vi "Process.vi"(8 "error in":errorcluster, 11 "DisplayWaveforms":refnum<class "DisplayWaveforms.lvclass">) -> (0 "error out":errorcluster, 3 "DisplayWaveforms out":refnum<class "DisplayWaveforms.lvclass">)   [LabVIEW 2020, in "DisplayWaveform.lvlib" / "DisplayWaveforms.lvclass"]
doc: "Displays all the waveforms using charts."
uses:
  DisplayWaveforms.lvclass
  C:/Program Files (x86)/National Instruments/LabVIEW 2020/vi.lib/JKI/JKI SMO/SMO/SMO.lvclass
  C:/Program Files (x86)/National Instruments/LabVIEW 2020/vi.lib/JKI/JKI SMO/SMO.UI/SMO.UI.lvclass
  <vilib>/JKI/JKI SMO/SMO/Typedefs/Parent Call--Enum.ctl
  Controller/TypeDefs/ChartParamsCluster.ctl
  DisplayWaveforms.lvclass/DisplayWaveforms.ctl
  <vilib>/JKI/JKI SMO/SMO.UI/SMO.UI.lvclass
  <vilib>/JKI/JKI SMO/SMO/SMO.lvclass
panel:
  out "Curr. Sense":dbl[][](graph)
  out "Amp. Volt.":dbl[][](graph)
  out "Ctrl. Eff":dbl[][](graph)
  out "Pos.":dbl[][](graph)
  out "Eddy Volt":dbl[][](graph)
  in  "------------- Registered Events -------------":bool
  in  "------------- Public API -------------":bool
  # "For instructions on how to use the JKI State Machine Objects, examples and video tutorials, visit:\nhttp://jki.net/state-machine-objects/\n\nJKI State Machine Objects™\nhttp://jki.net/state-machine-objects/\nCopyright (C) 2005-2015, JKI <info@jki.net>\nALL RIGHTS RESERVED"
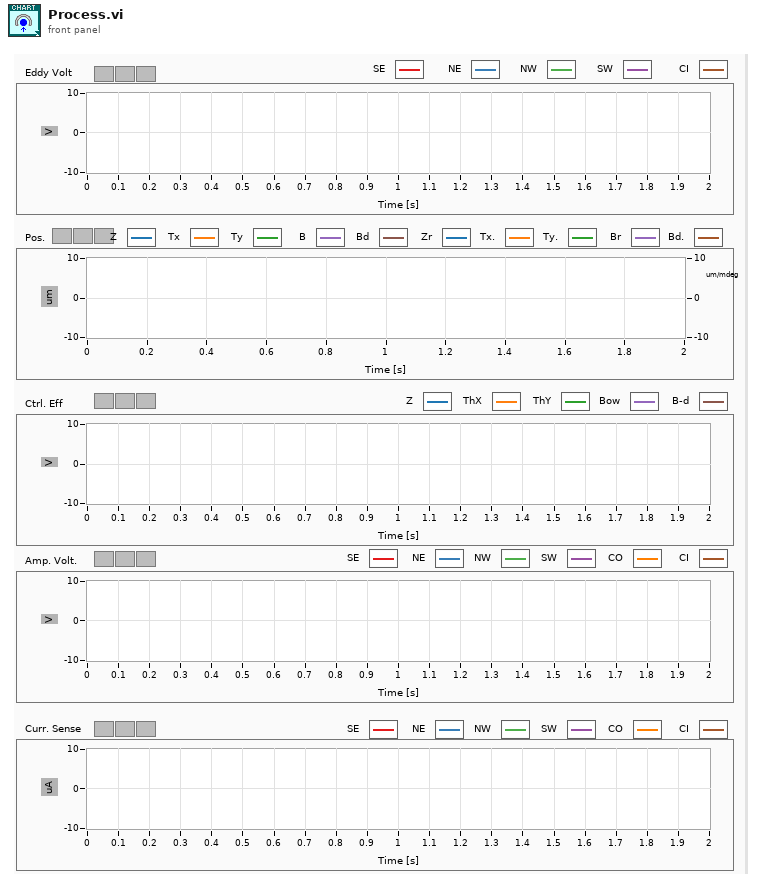
[diagram p1: front panel]
types:
  T1 = typedef "SMO.lvclass/Parent Call--Enum.ctl" = enum16{"Allows parent to run", "Does not request parent to run"}
  T2 = enum32{"invalid app kind", "Development System", "Run Time System", "Student Edition", "Embedded LabVIEW", "Evaluation", "Custom"}
  T3 = enum32{"Invalid", "Standard", "Closed", "Hidden", "Minimized", "Maximized"}
  T4 = typedef "ChartParamsCluster.ctl" = cluster{"Chart ScaleMultipliers":cluster{"WF Xscale Multiplier":dbl, "WF Yscale Multiplier":dbl[]}, "Coord Transform Multipliers":cluster{"Z-Multiplier":dbl, "Th-Multiplier":dbl}}
  T5 = cluster{"Core":cluster{"Current VI Reference":refnum<vi>, "Close Panel on Exit?":bool, "error":errorcluster}, "Self Reference":refnum<class "DisplayWaveforms.lvclass">, "bool":bool, "update chart?":bool, "ChartParams":T4, "Export Folder Path":path}
  T6 = cluster{"Current VI Reference":refnum<vi>, "Close Panel on Exit?":bool, "error":errorcluster}
  T7 = typedef "SMO.lvclass/Protected Events.ctl" = cluster{"StopProcesses":refnum<user-event>, "AbortProcesses":refnum<user-event>, "Config Changed":refnum<user-event>, "Dependency":refnum<user-event>}
  T8 = typedef "DisplayWaveform.lvlib/DisplayWaveforms.lvclass/ProtectedEvents--Cluster.ctl" = cluster{"Clear Chart":refnum<user-event>, "Pause Chart":refnum<user-event>, "Update Chart":refnum<user-event>, "Export Chart":refnum<user-event>, "Set ChartParams":refnum<user-event>}
  T9 = typedef "DisplayWaveform.lvlib/DisplayWaveforms.lvclass/Dependencies--Cluster.ctl" = cluster{"New Value":refnum<user-event>}
  T10 = typedef "imagedata.ctl" = cluster{"image type":i32, "image depth":i32, "image":u8[], "mask":u8[], "colors":u32[], "Rectangle":cluster{"left":i16, "top":i16, "right":i16, "bottom":i16}}
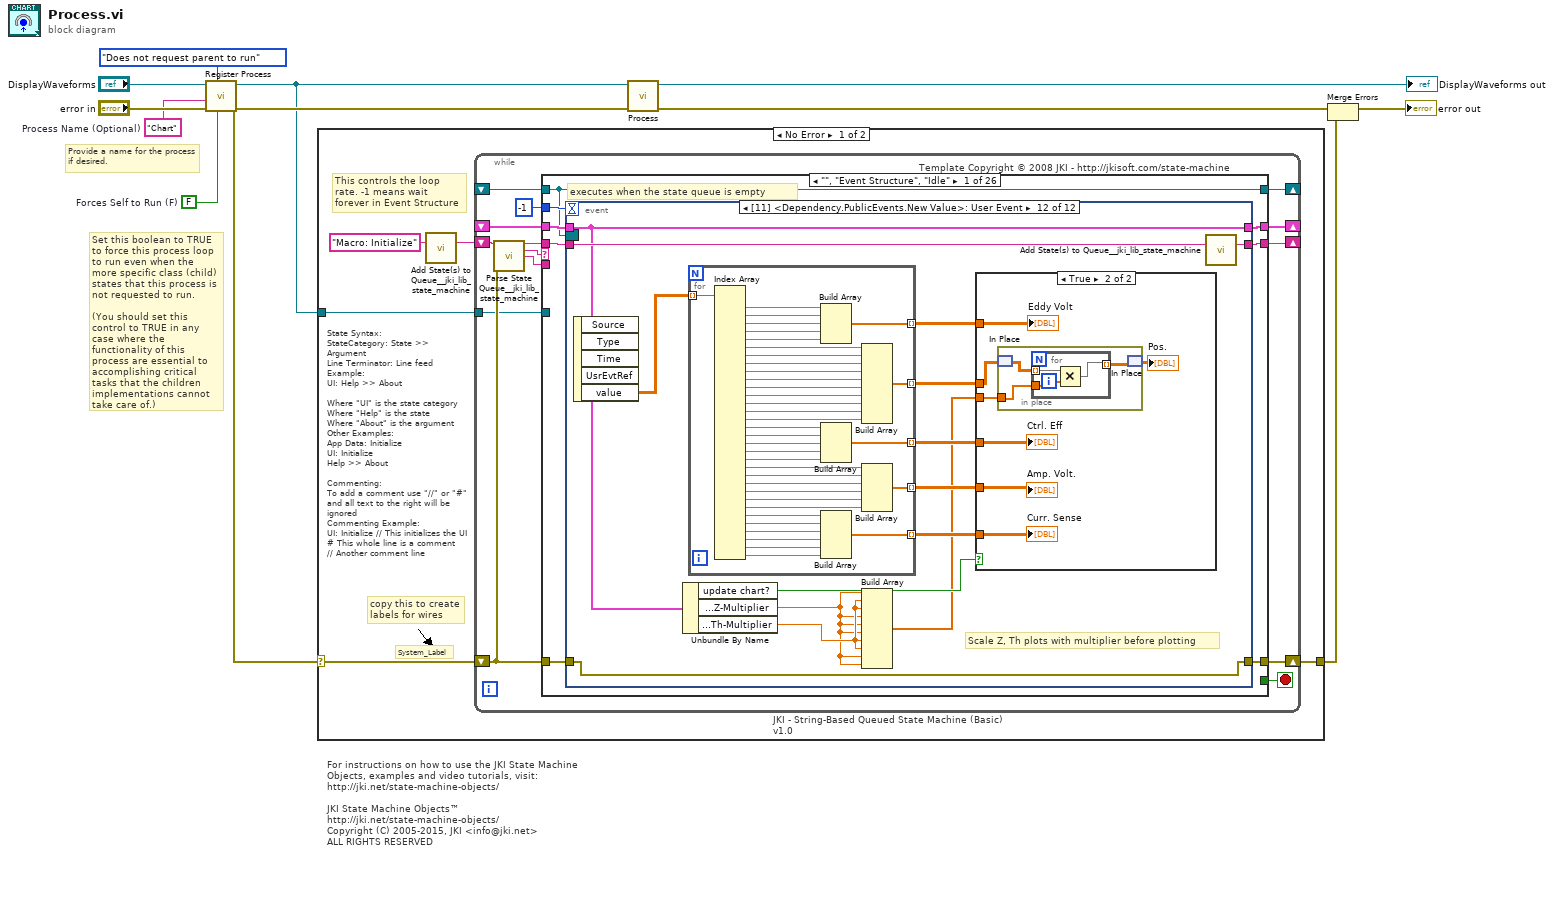
[diagram p0: block diagram]
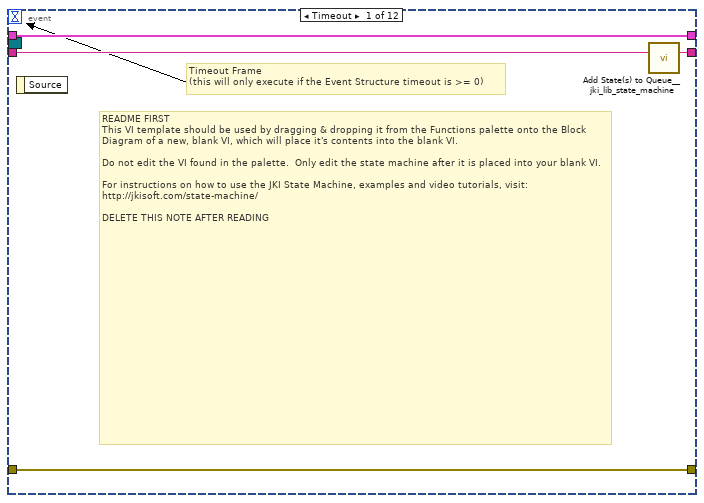
[diagram p2: hidden frame]
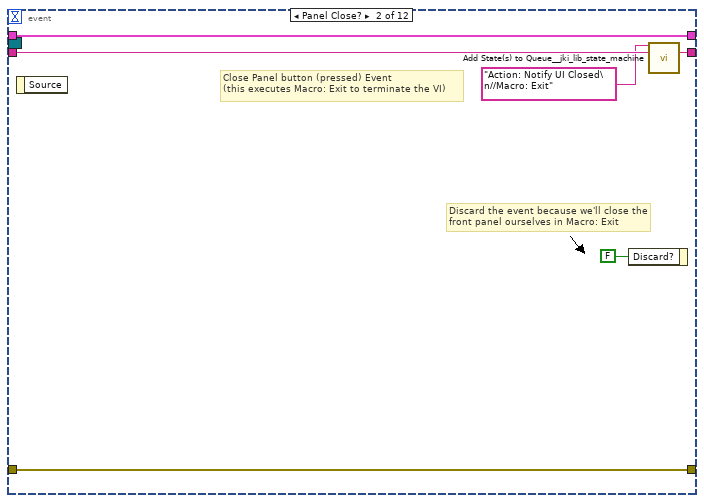
[diagram p3: hidden frame]
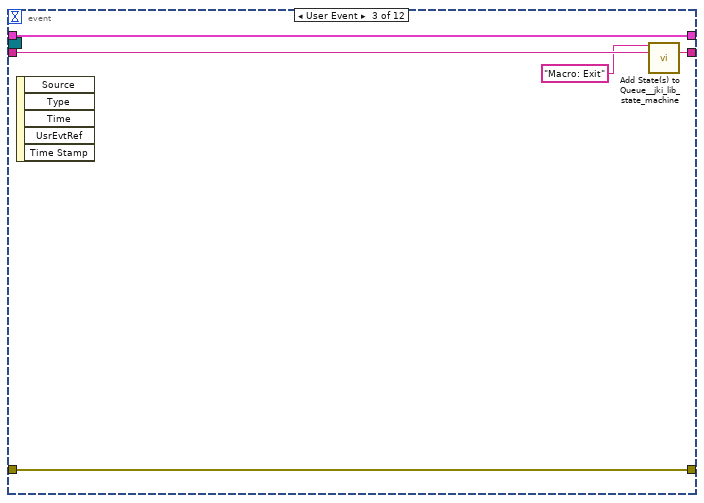
[diagram p4: hidden frame]
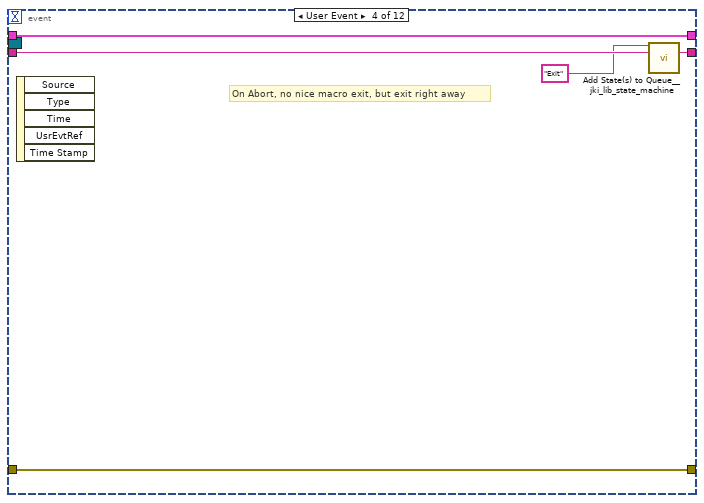
[diagram p5: hidden frame]
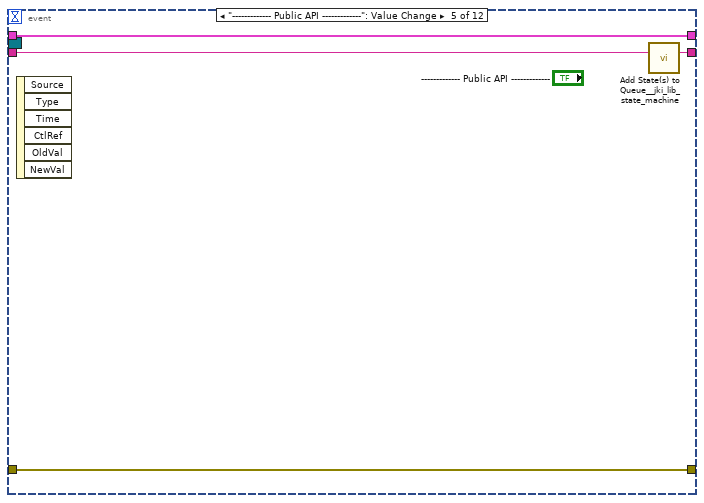
[diagram p6: hidden frame]
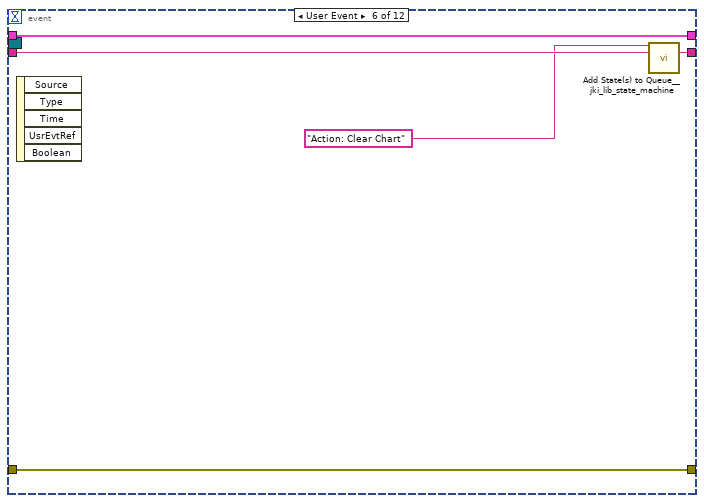
[diagram p7: hidden frame]
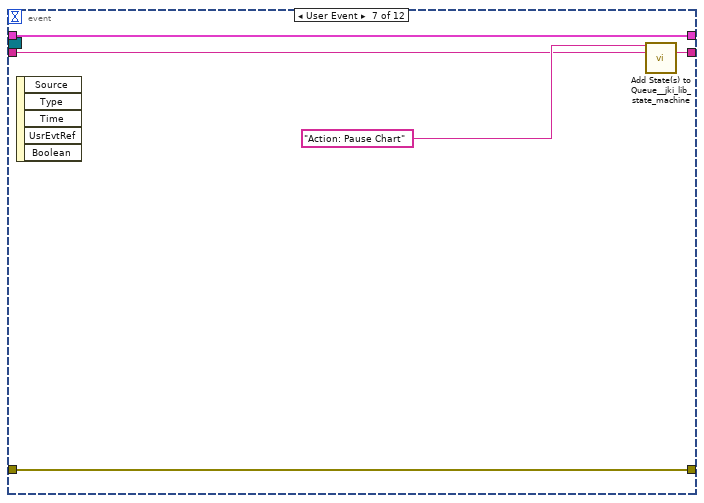
[diagram p8: hidden frame]
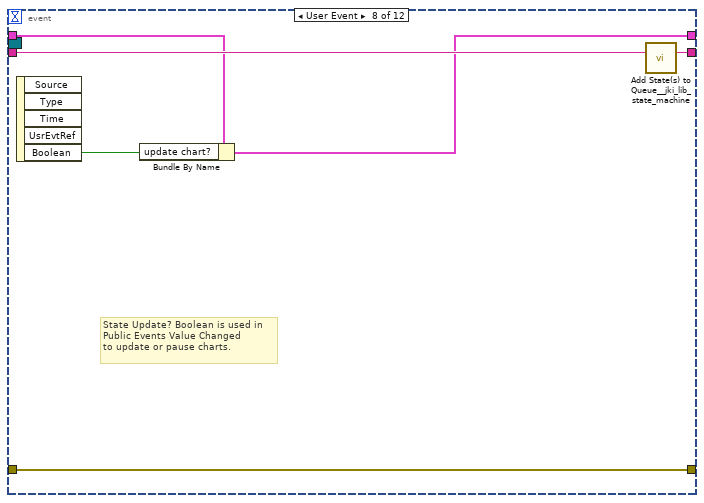
[diagram p9: hidden frame]
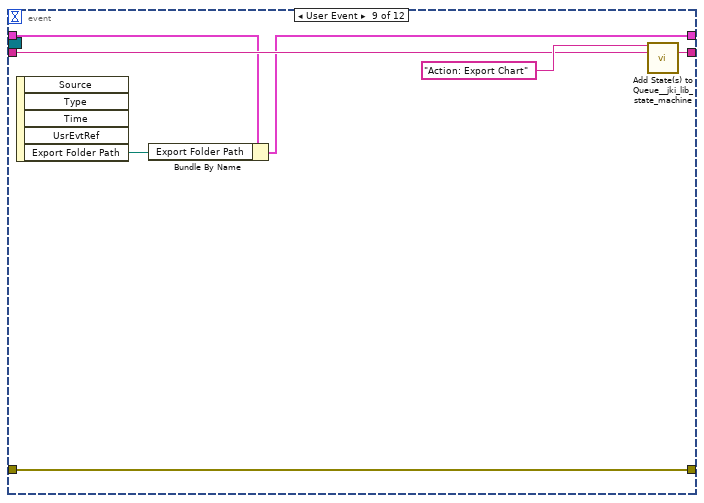
[diagram p10: hidden frame]
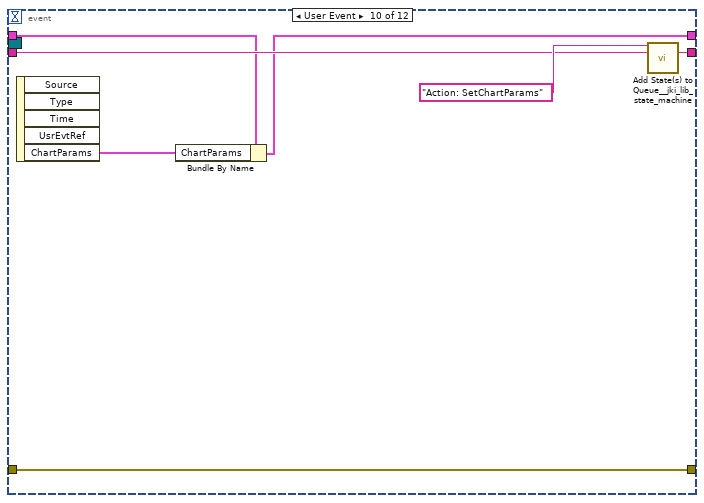
[diagram p11: hidden frame]
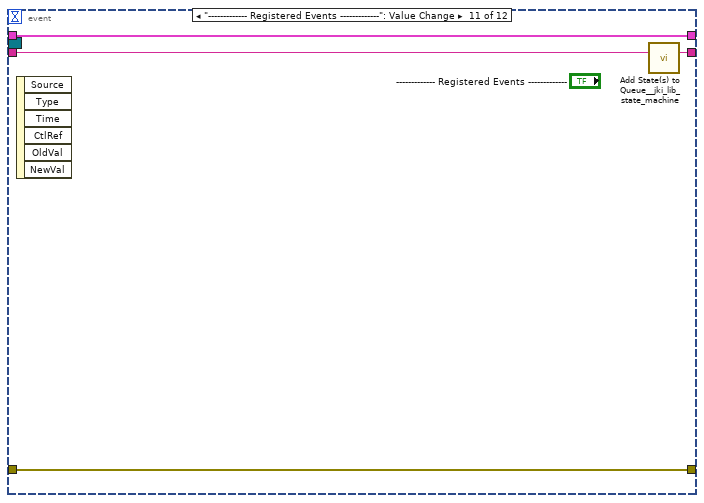
[diagram p12: hidden frame]
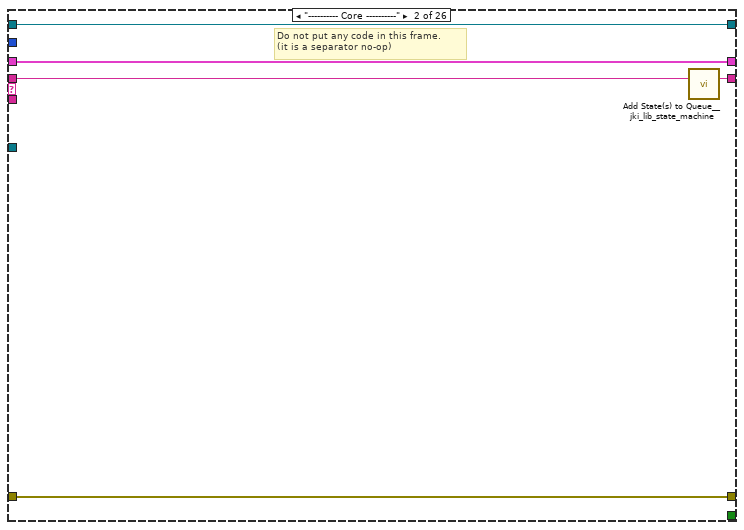
[diagram p14: hidden frame]
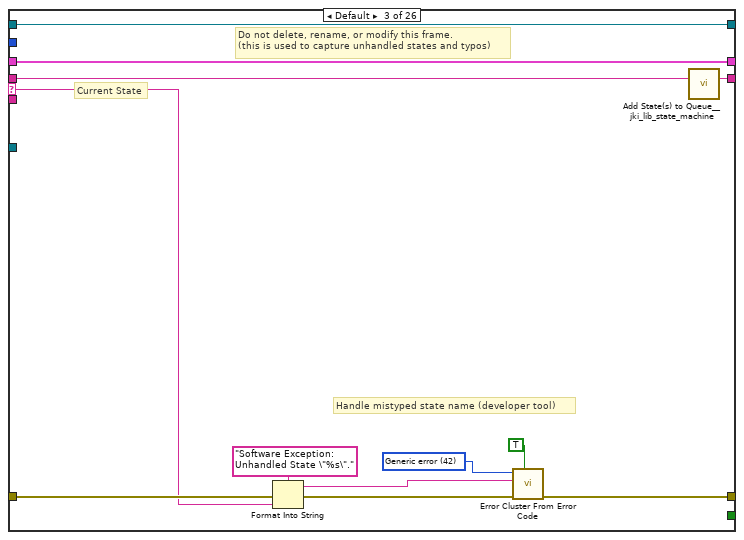
[diagram p15: hidden frame]
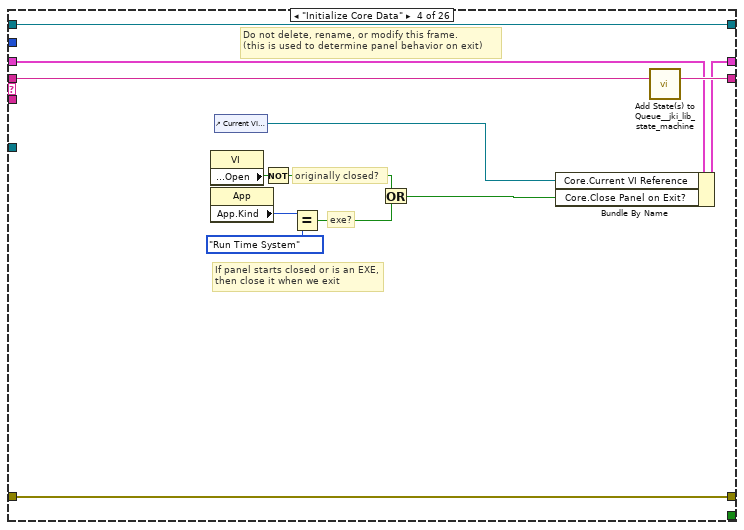
[diagram p16: hidden frame]
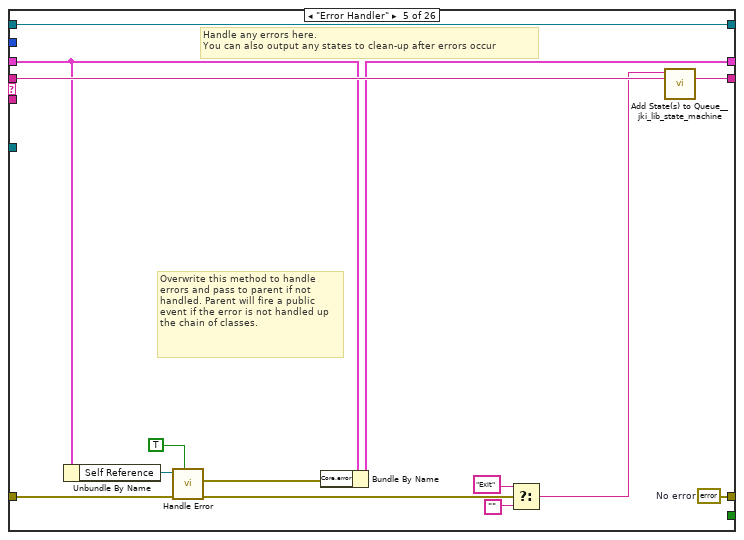
[diagram p17: hidden frame]
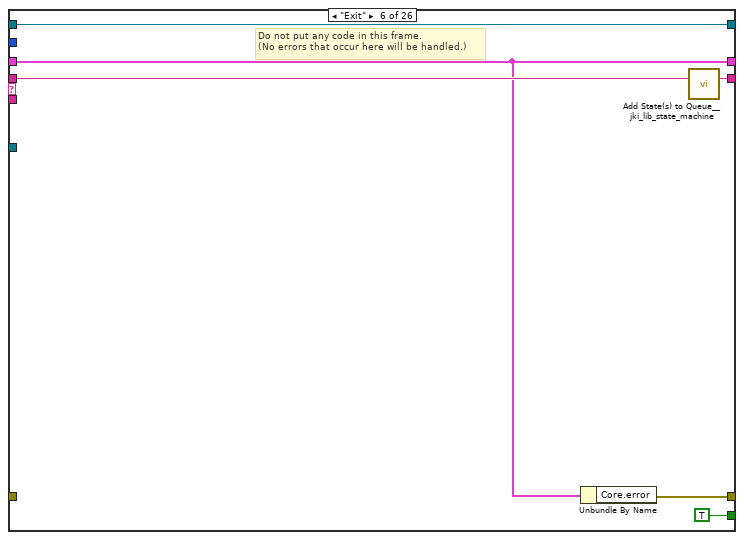
[diagram p18: hidden frame]
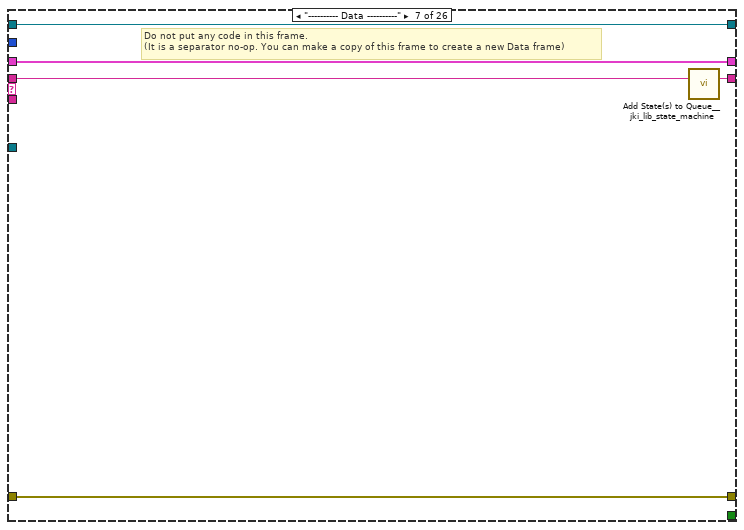
[diagram p19: hidden frame]
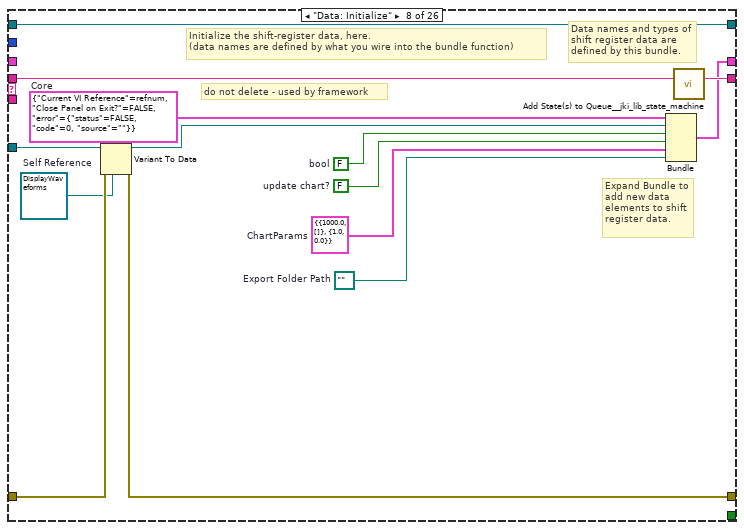
[diagram p20: hidden frame]
diagram:
  w2 = FALSE  # Forces Self to Run (F)
  w1 = "Chart"  # Process Name (Optional)
  # "Provide a name for the process\nif desired."
  # "Set this boolean to TRUE to force this process loop to run even when the more specific class (child) states that this process is not requested to run.\n\n(You should set this control to TRUE in any case where the functionality of this process are essential to accomplishing critical tasks that the children implementations cannot take care of.)"
  # "For instructions on how to use the JKI State Machine Objects, examples and video tutorials, visit:\nhttp://jki.net/state-machine-objects/\n\nJKI State Machine Objects™\nhttp://jki.net/state-machine-objects/\nCopyright (C) 2005-2015, JKI <info@jki.net>\nALL RIGHTS RESERVED"
  n1 = call <vilib>:"Register Process.vi"("Forces Self to Run (F)"=w2, "Parent Call"=Parent_Call--Enum."Does not request parent to run", "error in (no error)"="error in", "Process Name (optional)"=w1, "SMO"="DisplayWaveforms") -> ("error out"=w8:errorcluster, "SMO out"=w7:refnum<class "DisplayWaveforms.lvclass">)  [unwired: 5 in]
  n2 = case shown="No Error" w8 {
    selector: w8 -> [w13 w428]
    tunnel: w7 -> [w14 _]
    tunnel: [w12 w428] -> w4
    frame No Error {
      # "State Syntax:\nStateCategory: State >> Argument\nLine Terminator: Line feed\nExample:\nUI: Help >> About\n\nWhere \"UI\" is the state category\nWhere \"Help\" is the state\nWhere \"About\" is the argument\nOther Examples:\nApp Data: Initialize\nUI: Initialize\nHelp >> About\n\nCommenting:\nTo add a comment use \"//\" or \"#\" and all text to the right will be ignored\nCommenting Example:\nUI: Initialize // This initializes the UI\n# This whole line is a comment\n// Another comment line"
      # "copy this to create labels for wires"
      # "This controls the loop rate. -1 means wait forever in Event Structure"
      # "System_Label"
      n3 = call <vilib>:"Add State(s) to Queue__jki_lib_state_machine.vi"("State(s) in (\"\")"="Macro: Initialize") -> ("States Out"=w16:string)  [unwired: 14 in]
      n4 = while "JKI - String-Based Queued State Machine (Basic) v1.0" {
        shift-right: [w23] -> _
        shift-left: _ -> [w22]
        shift-right: [w26] -> w12
        shift-left: w13 -> [w20]
        shift-right: [w25] -> _
        shift-left: w16 -> [w27]
        tunnel: w14 -> [w19]
        shift-right: [w18] -> _
        shift-left: _ -> [w17]
        stop <- w24 stop-if-true
        # "Template Copyright © 2008 JKI - http://jkisoft.com/state-machine"
        n5 = call <vilib>:"Parse State Queue__jki_lib_state_machine.vi"("State Queue"=w27, "Error In (no error)"=w20) -> ("Remaining States"=w29:string, "Current State"=w30:string, "Arguments"=w28:string)  [unwired: 11 in]
        n6 = case shown="\"\", \"Event Structure\", \"Idle\"" w30 {
          selector: w30 -> [_ _ w168 _ _ _ _ _ _ _ _ _ _ _ _ _ _ _ _ _ _ _ _ _ _ _]
          tunnel: w29 -> [w38 w166 w172 w191 w205 w211 w216 w230 w237 w242 w255 w262 w278 w310 w319 w333 w338 w349 w354 w372 w384 w389 w396 w412 w420 w427]
          tunnel: w28 -> [_ _ _ _ _ _ _ _ _ _ _ w256 w272 _ _ _ _ _ _ _ _ _ _ _ _ _]
          tunnel: w22 -> [w36 w163 w170 w182 w194 w207 w213 _ w232 w239 w251 w260 w274 w307 w315 w324 w335 w346 w351 w370 w382 w387 w393 w409 w417 w423]
          tunnel: [w35 w164 w174 w188 w196 w206 w214 w225 w233 w240 w253 w257 w275 w308 w317 w331 w336 w340 w352 w367 w380 w385 w391 w398 w415 w421] -> w26
          tunnel: w20 -> [w34 w164 w173 w188 w201 _ w214 w226 w234 w240 w253 w258 w276 w308 w317 w331 w336 w341 w352 w363 w380 w385 w392 w408 w416 w422]
          tunnel: [w37 w165 w171 w190 w204 w210 w215 w229 w236 w241 w254 w261 w277 w309 w318 w332 w337 w348 w353 w371 w383 w388 w395 w411 w419 w426] -> w25
          tunnel: [_ _ _ _ _ TRUE _ _ _ _ _ _ _ _ _ _ _ _ _ _ _ _ _ _ _ _] -> w24
          tunnel: [w33 w163 w170 w189 w193 w207 w213 w228 w232 w239 w250 w260 w274 w307 w315 w324 w335 w346 w351 w370 w382 w387 w393 w409 w417 w423] -> w23
          tunnel: -1 ("Timeout") -> [w32 _ _ _ _ _ _ _ _ _ _ _ _ _ _ _ _ _ _ _ _ _ _ _ _ _]
          tunnel: w19 -> [_ _ _ _ _ _ _ w223 _ _ _ _ _ _ _ _ _ _ _ _ _ _ _ _ _ _]
          tunnel: [w31 w162 w167 w179 w203 w208 w212 w221 w231 w238 w252 w259 w271 w306 w316 w325 w334 w347 w350 w369 w381 w386 w394 w410 w418 w425] -> w18
          tunnel: w17 -> [w31 w162 w167 w179 w203 w208 w212 w221 w231 w238 w252 w259 w271 w306 w316 w325 w334 w347 w350 _ w381 w386 w394 w410 w418 w425]
          frame "", "Event Structure", "Idle" {
            # "executes when the state queue is empty"
            n7 = event shown="[11] <Dependency.PublicEvents.New Value>: User Event" {
              selector: w31 -> [_ _ _ _ _ _ _ _ _ _ _ _]
              dyn-events: _ -> [_ _ _ _ _ _ _ _ _ _ _ _]
              timeout: w32 -> [_ _ _ _ _ _ _ _ _ _ _ _]
              tunnel: w38 -> [w42 w48 w53 w58 w62 w67 w71 w78 w84 w91 w96 w110]
              tunnel: [w41 w47 w52 w57 w61 w66 w69 w77 w83 w90 w95 w109] -> w37
              tunnel: w36 -> [w39 w44 w50 w55 w59 w64 w70 w75 w81 w88 w93 w101]
              tunnel: [w40 w43 w51 w56 w60 w65 w68 w76 w82 w89 w94 w108] -> w35
              tunnel: w34 -> [w40 w43 w51 w56 w60 w65 w68 w76 w82 w89 w94 w108]
              tunnel: [w39 w44 w50 w55 w59 w64 w70 w73 w79 w86 w93 w101] -> w33
              event Timeout {
                # "README FIRST\nThis VI template should be used by dragging & dropping it from the Functions palette onto the Block Diagram of a new, blank VI, which will place it's contents into the blank VI.\n\nDo not edit the VI found in the palette.  Only edit the state machine after it is placed into your blank VI.\n\nFor instructions on how to use the JKI State Machine, examples and video tutorials, visit:\nhttp://jkisoft.com/state-machine/\n\nDELETE THIS NOTE AFTER READING"
                # "Timeout Frame\n(this will only execute if the Event Structure timeout is >= 0)"
                n8 = event-data() -> ()  [unwired: 1 in, 1 out]
                n9 = call <vilib>:"Add State(s) to Queue__jki_lib_state_machine.vi"("State(s) in (\"\")"=w42) -> ("States Out"=w41:string)  [unwired: 14 in]
              }
              event Panel Close? {
                # "Discard the event because we'll close the front panel ourselves in Macro: Exit"
                # "Close Panel button (pressed) Event\n(this executes Macro: Exit to terminate the VI)"
                n10 = event-data() -> ()  [unwired: 1 in, 1 out]
                n11 = event-data("Discard?"=FALSE) -> ()  [unwired: 1 in, 1 out]
                n12 = call <vilib>:"Add State(s) to Queue__jki_lib_state_machine.vi"("State(s) in Front (\"\")"="Action: Notify UI Closed\n//Macro: Exit", "State(s) in (\"\")"=w48) -> ("States Out"=w47:string)  [unwired: 13 in]
              }
              event User Event {
                n13 = event-data() -> ()  [unwired: 1 in, 5 out]
                n14 = call <vilib>:"Add State(s) to Queue__jki_lib_state_machine.vi"("State(s) in Front (\"\")"="Macro: Exit", "State(s) in (\"\")"=w53) -> ("States Out"=w52:string)  [unwired: 13 in]
              }
              event User Event {
                # "On Abort, no nice macro exit, but exit right away"
                n15 = event-data() -> ()  [unwired: 1 in, 5 out]
                n16 = call <vilib>:"Add State(s) to Queue__jki_lib_state_machine.vi"("State(s) in Front (\"\")"="Exit", "State(s) in (\"\")"=w58) -> ("States Out"=w57:string)  [unwired: 13 in]
              }
              event "------------- Public API -------------": Value Change {
                n17 = event-data() -> ()  [unwired: 1 in, 6 out]
                n18 = call <vilib>:"Add State(s) to Queue__jki_lib_state_machine.vi"("State(s) in (\"\")"=w62) -> ("States Out"=w61:string)  [unwired: 14 in]
              }
              event User Event {
                n19 = event-data() -> ()  [unwired: 1 in, 5 out]
                n20 = call <vilib>:"Add State(s) to Queue__jki_lib_state_machine.vi"("State(s) in Front (\"\")"="Action: Clear Chart", "State(s) in (\"\")"=w67) -> ("States Out"=w66:string)  [unwired: 13 in]
              }
              event User Event {
                n21 = event-data() -> ()  [unwired: 1 in, 5 out]
                n22 = call <vilib>:"Add State(s) to Queue__jki_lib_state_machine.vi"("State(s) in Front (\"\")"="Action: Pause Chart", "State(s) in (\"\")"=w71) -> ("States Out"=w69:string)  [unwired: 13 in]
              }
              event User Event {
                # "State Update? Boolean is used in \nPublic Events Value Changed \nto update or pause charts."
                n23 = event-data() -> ("Boolean"=w74:bool)  [unwired: 1 in, 4 out]
                n24 = Bundle By Name(cluster=w75, "update chart?"=w74) -> (w73:T5)
                n25 = call <vilib>:"Add State(s) to Queue__jki_lib_state_machine.vi"("State(s) in (\"\")"=w78) -> ("States Out"=w77:string)  [unwired: 14 in]
              }
              event User Event {
                n26 = event-data() -> ("Export Folder Path"=w80:path)  [unwired: 1 in, 4 out]
                n27 = Bundle By Name(cluster=w81, "Export Folder Path"=w80) -> (w79:T5)
                n28 = call <vilib>:"Add State(s) to Queue__jki_lib_state_machine.vi"("State(s) in Front (\"\")"="Action: Export Chart", "State(s) in (\"\")"=w84) -> ("States Out"=w83:string)  [unwired: 13 in]
              }
              event User Event {
                n29 = event-data() -> ("ChartParams"=w87:T4)  [unwired: 1 in, 4 out]
                n30 = Bundle By Name(cluster=w88, "ChartParams"=w87) -> (w86:T5)
                n31 = call <vilib>:"Add State(s) to Queue__jki_lib_state_machine.vi"("State(s) in Front (\"\")"="Action: SetChartParams", "State(s) in (\"\")"=w91) -> ("States Out"=w90:string)  [unwired: 13 in]
              }
              event "------------- Registered Events -------------": Value Change {
                n32 = event-data() -> ()  [unwired: 1 in, 6 out]
                n33 = call <vilib>:"Add State(s) to Queue__jki_lib_state_machine.vi"("State(s) in (\"\")"=w96) -> ("States Out"=w95:string)  [unwired: 14 in]
              }
              event User Event {
                # "Scale Z, Th plots with multiplier before plotting"
                n34 = event-data() -> ("value"=w107:dbl[][])  [unwired: 1 in, 4 out]
                n35 = Unbundle By Name(w101) -> ("update chart?"=w100:bool, "ChartParams.Coord Transform Multipliers.Z-Multiplier"=w97:dbl, "ChartParams.Coord Transform Multipliers.Th-Multiplier"=w98:dbl)
                n36 = for {
                  tunnel: w107 -> [w161] mode=indexing
                  tunnel: [w160] -> w106 mode=indexing
                  tunnel: [w159] -> w105 mode=indexing
                  tunnel: [w158] -> w104 mode=indexing
                  tunnel: [w157] -> w103 mode=indexing
                  tunnel: [w156] -> w102 mode=indexing
                  n37 = Index Array(array=w161) -> (element #1=w155:dbl, element #2=w154:dbl, element #3=w153:dbl, element #4=w152:dbl, element #5=w151:dbl, element #6=w150:dbl, element #7=w149:dbl, element #8=w148:dbl, element #9=w147:dbl, element #10=w146:dbl, element #11=w145:dbl, element #12=w144:dbl, element #13=w143:dbl, element #14=w142:dbl, element #15=w141:dbl, element #16=w140:dbl, element #17=w139:dbl, element #18=w138:dbl, element #19=w137:dbl, element #20=w136:dbl, element #21=w135:dbl, element #22=w134:dbl, element #23=w133:dbl, element #24=w132:dbl, element #25=w131:dbl, element #26=w130:dbl, element #27=w129:dbl, element #28=w128:dbl, element #29=w127:dbl, element #30=w126:dbl, element #31=w125:dbl, element #32=w124:dbl)  [unwired: 32 in]
                  n38 = Build Array(w155, w154, w153, w152, w151) -> (w160:dbl[])
                  n39 = Build Array(w140, w139, w138, w137, w136) -> (w158:dbl[])
                  n40 = Build Array(w129, w128, w127, w126, w125, w124) -> (w156:dbl[])
                  n41 = Build Array(w150, w149, w148, w147, w146, w145, w144, w143, w142, w141) -> (w159:dbl[])
                  n42 = Build Array(w135, w134, w133, w132, w131, w130) -> (w157:dbl[])
                }
                n43 = Build Array(w97, w98, w98, w97, w97, w97, w98, w98, w97, w97) -> (w99:dbl[])
                n44 = case shown="True" w100 {
                  tunnel: w106 -> [_ w117]
                  tunnel: w105 -> [_ w113]
                  tunnel: w104 -> [_ w116]
                  tunnel: w103 -> [_ w115]
                  tunnel: w102 -> [_ w114]
                  tunnel: w99 -> [_ w111]
                  frame False {
                  }
                  frame True {
                    n45 = in-place {
                      in-place-border: w111 -> [w119]
                      n46 = in-place-match #1(w113) -> (w120:dbl[][])
                      n47 = for {
                        tunnel: w120 -> [w123] mode=indexing
                        tunnel: w119 -> [w122]
                        tunnel: [w121] -> w118 mode=indexing
                        n48 = Multiply(x=w123, y=w122) -> (x*y=w121:dbl[])
                      }
                      n49 = in-place-match #1(w118) -> (→"Pos.":dbl[][])
                    }
                    "Eddy Volt" <- w117
                    "Curr. Sense" <- w114
                    "Amp. Volt." <- w115
                    "Ctrl. Eff" <- w116
                  }
                }
                n50 = call <vilib>:"Add State(s) to Queue__jki_lib_state_machine.vi"("State(s) in (\"\")"=w110) -> ("States Out"=w109:string)  [unwired: 14 in]
              }
            }
          }
          frame "---------- Core ----------" {
            # "Do not put any code in this frame.\n(it is a separator no-op)"
            n51 = call <vilib>:"Add State(s) to Queue__jki_lib_state_machine.vi"("State(s) in (\"\")"=w166) -> ("States Out"=w165:string)  [unwired: 14 in]
          }
          frame Default {
            w177 = 42 items=["No error", "Argument error", "Memory is full", "Out of zone", "End of file", "File already open", "Generic file I/O error", "File not found", "File permission error", "Disk is full", "Duplicate path", "Too many files open", "System feature not enabled", "Resource file not found", "Cannot add resource", "Resource not found", "Image not found", "Image memory error", "Pen does not exist", "Config type invalid", "Config token not found", "Config parse error", "Config memory error", "Bad external code format", "Bad external code offset", "External code not present", "Null window", "Destroy window error", "Null menu", "Print aborted", "Bad print record", "Print driver error", "Windows error during printing", "Memory error during printing", "Print dialog error", "Generic print error", "Invalid device refnum", "Device not found", "Device parameter error", "Device unit error", "Cannot open device", "Device call aborted", "Generic error", "Cancelled by user", "Object ID too low", "Object ID too high", "Object not in heap", "Unknown heap", "Unknown object (invalid DefProc)", "Unknown object (DefProc not in table)", "Message out of range", "Invalid (null) method", "Unknown message", "Manager call not supported", "Bad address", "Network operation in progress", "Network operation timed out", "Connection is busy", "Network attribute not supported", "Network error", "Address in use", "System out of memory", "Connection aborted", "Connection refused", "Not connected", "Already connected", "Connection closed", "Initialization error (interapplication manager)", "Bad occurrence", "Wait on unbound occurrence handler", "Occurrence queue overflow", "Datalog type conflict", "Unused", "Unrecognized type (interapplication manager)", "Memory corrupt", "Failed to make temporary DLL", "Old CIN version", "Drag socket not found", "Failed to load drop-object", "Failed to register OLE object", "Failed to release OLE object", "Format specifier type mismatch", "Unknown format specifier", "Too few format specifiers", "Too many format specifiers", "Scan failed", "Newer CIN version", "Error converting to variant", "Runtime menu error", "Password tampered", "Variant attribute not found", "Incompatible variant data type", "Event data is not available", "Event Store is not present", "Occurrence is not found", "Event Queue is not created", "Event info is not available", "Refnum passed is NULL", "Error retrieving Class GUID", "Error retrieving CoClass GUID", "Error retrieving TypeLib GUID.", "Bad built application magic bytes.", "Specific driver is different from the specific driver associated with the Logical Name.", "There is no session opened to the class driver.", "Max Error", "MAX - Error with config objects", "MAX - Error loading configuration", "MAX - Group not supported"]
            # "Current State"
            # "Do not delete, rename, or modify this frame.\n(this is used to capture unhandled states and typos)"
            # "Handle mistyped state name (developer tool)"
            n52 = Format Into String(format string="Software Exception: Unhandled State \"%s\"." ("message"), error in=w173, w168) -> (resulting string=w176:string, error out=w175:errorcluster)  [unwired: 1 in]
            n53 = call <vilib>:"Error Cluster From Error Code.vi"("show call chain? (False)"=TRUE, "error in (no error)"=w175, "error message (\"\")"=w176, "error code (0)"=w177) -> ("error out"=w174:errorcluster)  [unwired: 5 in]
            n54 = call <vilib>:"Add State(s) to Queue__jki_lib_state_machine.vi"("State(s) in (\"\")"=w172) -> ("States Out"=w171:string)  [unwired: 14 in]
          }
          frame "Initialize Core Data" {
            # "Do not delete, rename, or modify this frame.\n(this is used to determine panel behavior on exit)"
            # "originally closed?"
            # "exe?"
            # "If panel starts closed or is an EXE, then close it when we exit"
            n55 = property class="VI"() -> ("Front Panel.Open"=w187:bool)  [unwired: 2 in, 2 out]
            n56 = property class="App"() -> ("App.Kind"=w186:T2)  [unwired: 2 in, 2 out]
            n57 = control-ref of="Current VI Reference"() -> (w180:refnum<vi>)
            n58 = Not(x=w187) -> (.not. x?=w184:bool)
            n59 = Equal?(x=w186, y=T2."Run Time System" ("Application:Kind")) -> (x = y?=w183:bool)
            n60 = Or(x=w184, y=w183) -> (x .or. y?=w181:bool)
            n61 = Bundle By Name(cluster=w182, "Core.Current VI Reference"=w180, "Core.Close Panel on Exit?"=w181) -> (w189:T5)
            n62 = call <vilib>:"Add State(s) to Queue__jki_lib_state_machine.vi"("State(s) in (\"\")"=w191) -> ("States Out"=w190:string)  [unwired: 14 in]
          }
          frame "Error Handler" {
            w196 = errorcluster {"status"=FALSE, "code"=0, "source"=""}  # No error
            # "Overwrite this method to handle errors and pass to parent if not handled. Parent will fire a public event if the error is not handled up the chain of classes."
            # "Handle any errors here.\nYou can also output any states to clean-up after errors occur"
            n63 = Unbundle By Name(w194) -> ("Self Reference"=w202:refnum<class "DisplayWaveforms.lvclass">)
            n64 = call-dynamic "Handle Error.vi"("Stop on Unhandled Error (T)"=TRUE, "error in"=w201, "SMO"=w202) -> ("handling error"=w197:errorcluster, "Unhandled error"=w195:errorcluster)  [unwired: 6 in, 1 out]
            n65 = Bundle By Name(cluster=w194, "Core.error"=w195) -> (w193:T5)
            n66 = Select(t="Exit", s=w197, f="") -> (s? t:f=w198:string)
            n67 = call <vilib>:"Add State(s) to Queue__jki_lib_state_machine.vi"("State(s) in Front (\"\")"=w198, "State(s) in (\"\")"=w205) -> ("States Out"=w204:string)  [unwired: 13 in]
          }
          frame "Exit" {
            # "Do not put any code in this frame.\n(No errors that occur here will be handled.)"
            n68 = Unbundle By Name(w207) -> ("Core.error"=w206:errorcluster)
            n69 = call <vilib>:"Add State(s) to Queue__jki_lib_state_machine.vi"("State(s) in (\"\")"=w211) -> ("States Out"=w210:string)  [unwired: 14 in]
          }
          frame "---------- Data ----------" {
            # "Do not put any code in this frame.\n(It is a separator no-op. You can make a copy of this frame to create a new Data frame)"
            n70 = call <vilib>:"Add State(s) to Queue__jki_lib_state_machine.vi"("State(s) in (\"\")"=w216) -> ("States Out"=w215:string)  [unwired: 14 in]
          }
          frame "Data: Initialize" {
            w217 = path ""  # Export Folder Path
            w218 = T4 {"Chart ScaleMultipliers"={"WF Xscale Multiplier"=1000.0, "WF Yscale Multiplier"=[]}, "Coord Transform Multipliers"={"Z-Multiplier"=1.0, "Th-Multiplier"=0.0}}  # ChartParams
            w219 = FALSE  # update chart?
            w220 = T6 {"Current VI Reference"=refnum, "Close Panel on Exit?"=FALSE, "error"={"status"=FALSE, "code"=0, "source"=""}}  # Core
            w224 = refnum<class "DisplayWaveforms.lvclass"> refnum  # Self Reference
            w227 = FALSE  # bool
            # "do not delete - used by framework"
            # "Expand Bundle to add new data elements to shift register data."
            # "Data names and types of shift register data are defined by this bundle."
            # "Initialize the shift-register data, here.\n(data names are defined by what you wire into the bundle function)"
            n71 = Variant To Data(error in=w226, type=w224, Variant=w223) -> (data=w222:refnum<class "DisplayWaveforms.lvclass">, error out=w225:errorcluster)
            n72 = Bundle("Core"=w220, "Self Reference"=w222, "bool"=w227, "update chart?"=w219, "ChartParams"=w218, "Export Folder Path"=w217) -> (w228:T5)  [unwired: 1 in]
            n73 = call <vilib>:"Add State(s) to Queue__jki_lib_state_machine.vi"("State(s) in (\"\")"=w230) -> ("States Out"=w229:string)  [unwired: 14 in]
          }
          frame "Data: Cleanup" {
            # "Cleanup any data and references, here.\n(this is called automatically, by the Macro: Exit)"
            n74 = Unbundle By Name(w232) -> ("Core.Current VI Reference"=w235:refnum<vi>)
            n75 = Close Reference(reference=w235, error in (no error)=w234) -> (error out=w233:errorcluster)
            n76 = call <vilib>:"Add State(s) to Queue__jki_lib_state_machine.vi"("State(s) in (\"\")"=w237) -> ("States Out"=w236:string)  [unwired: 14 in]
          }
          frame "---------- UI ----------" {
            # "Do not put any code in this frame.\n(It is a separator no-op. You can make a copy of this frame to create a new UI frame)"
            n77 = call <vilib>:"Add State(s) to Queue__jki_lib_state_machine.vi"("State(s) in (\"\")"=w242) -> ("States Out"=w241:string)  [unwired: 14 in]
          }
          frame "UI: Initialize" {
            # "Initialize the User Interface, here.\n(this is called automatically, by the Macro: Init)"
            n78 = control-ref of="Eddy Volt"() -> (w247:refnum<vi>)
            n79 = control-ref of="Pos."() -> (w246:refnum<vi>)
            n80 = control-ref of="Ctrl. Eff"() -> (w245:refnum<vi>)
            n81 = control-ref of="Amp. Volt."() -> (w244:refnum<vi>)
            n82 = control-ref of="Curr. Sense"() -> (w243:refnum<vi>)
            n83 = Unbundle By Name(w251) -> ("Self Reference"=w249:refnum<class "DisplayWaveforms.lvclass">)
            n84 = Bundle By Name(cluster=w249, "WFChart Refnum"=w247, "WFChart Refnum 2"=w246, "WFChart Refnum 3"=w245, "WFChart Refnum 4"=w244, "WFChart Refnum 5"=w243) -> (w248:refnum<class "DisplayWaveforms.lvclass">)
            n85 = Bundle By Name(cluster=w251, "Self Reference"=w248) -> (w250:T5)
            n86 = call <vilib>:"Add State(s) to Queue__jki_lib_state_machine.vi"("State(s) in (\"\")"=w255) -> ("States Out"=w254:string)  [unwired: 14 in]
          }
          frame "UI: Cursor Set" {
            # "Argument"
            # "Initialize the User Interface, here.\n(this is called automatically, by the Macro: Init)"
            n87 = disable-structure shown="Default" {
              disable-tunnel: w258 -> [w263 w266]
              disable-tunnel: [w263 w265] -> w257
              disable-tunnel: w256 -> [_ w264]
              frame condition #0 {
              }
              frame condition #1 (active) {
                n88 = case shown="\"Idle\", Default" w264 {
                  tunnel: w266 -> [w268 w270]
                  tunnel: [w267 w269] -> w265
                  frame "Idle", Default {
                    n89 = call <vilib>:"Unset Busy.vi"("error in (no error)"=w268) -> ("error out"=w267:errorcluster)  [unwired: 10 in]
                  }
                  frame "Busy" {
                    n90 = call <vilib>:"Set Busy.vi"("error in (no error)"=w270) -> ("error out"=w269:errorcluster)  [unwired: 9 in, 1 out]
                  }
                }
              }
            }
            n91 = call <vilib>:"Add State(s) to Queue__jki_lib_state_machine.vi"("State(s) in (\"\")"=w262) -> ("States Out"=w261:string)  [unwired: 14 in]
          }
          frame "UI: Front Panel State" {
            # "Argument"
            # "Set Front Panel Open or Closed\n(Usage: \"UI: Front Panel State >> Open|Close\")"
            n92 = Unbundle By Name(w274) -> ("Core.Current VI Reference"=w273:refnum<vi>)
            n93 = disable-structure shown="Default" {
              disable-tunnel: w276 -> [w282 w305]
              disable-tunnel: [w281 w305] -> w275
              disable-tunnel: w273 -> [w280 _]
              disable-tunnel: w272 -> [w279 _]
              frame condition #0 (active) {
                n94 = case shown="\"Close\"" w279 {
                  tunnel: w282 -> [w286 w299]
                  tunnel: [w288 w300] -> w281
                  tunnel: w280 -> [w287 w297]
                  frame "Open", Default {
                    n95 = property class="VI"(reference=w287, error in=w286) -> (reference out=w284:refnum<vi>, error out=w285:errorcluster, "FP.State"=w283:T3)
                    n96 = case shown="\"Closed\"" w283 {
                      tunnel: [w291 w294] -> w288
                      tunnel: w285 -> [w290 w294]
                      tunnel: w284 -> [w289 _]
                      frame "Closed" {
                        n97 = invoke class="VI" method="FP.Open"(reference=w289, error in=w290, "Activate"=TRUE, "State"=T3."Standard") -> (error out=w291:errorcluster)  [unwired: 1 in, 4 out]
                      }
                      frame Default {
                      }
                    }
                  }
                  frame "Close" {
                    n98 = property class="VI"(reference=w297, error in=w299) -> (reference out=w296:refnum<vi>, error out=w298:errorcluster, "FP.State"=w295:T3)
                    n99 = case shown="Default" w295 {
                      tunnel: [w301 w304] -> w300
                      tunnel: w298 -> [w301 w303]
                      tunnel: w296 -> [_ w302]
                      frame "Invalid", "Closed" {
                      }
                      frame Default {
                        n100 = invoke class="VI" method="FP.Close"(reference=w302, error in=w303) -> (error out=w304:errorcluster)  [unwired: 1 in, 2 out]
                      }
                    }
                  }
                }
              }
              frame condition #1 {
              }
            }
            n101 = call <vilib>:"Add State(s) to Queue__jki_lib_state_machine.vi"("State(s) in (\"\")"=w278) -> ("States Out"=w277:string)  [unwired: 14 in]
          }
          frame "---------- Macro ----------" {
            # "Do not put any code in this frame.\n(It is a separator no-op. You can make a copy of this frame to create a new Macro frame)"
            n102 = call <vilib>:"Add State(s) to Queue__jki_lib_state_machine.vi"("State(s) in (\"\")"=w310) -> ("States Out"=w309:string)  [unwired: 14 in]
          }
          frame "Macro: Initialize" {
            w313 = "UI: Initialize\n//UI: Front Panel State >> Open"  # UI: Initialize //UI: Front Panel State >> Open
            # "Initialization Macro\n(This is called once, when the VI starts)"
            n103 = call <vilib>:"Add State(s) to Queue__jki_lib_state_machine.vi"("State(s) in Front (\"\")"="Data: Initialize\nInitialize Core Data\nEvents: Register", "State(s) in (\"\")"="Process: Sync", "State(s) at Back (\"\")"=w313) -> ("States Out"=w312:string)  [unwired: 12 in]
            n104 = call <vilib>:"Add State(s) to Queue__jki_lib_state_machine.vi"("State(s) in Front (\"\")"=w312, "State(s) in (\"\")"=w319) -> ("States Out"=w318:string)  [unwired: 13 in]
          }
          frame "Macro: Exit" {
            # "Exit Macro\n(This is called once, when the VI exits)"
            n105 = Unbundle By Name(w324) -> ("Core.Close Panel on Exit?"=w330:bool)
            n106 = Select(t="//UI: Front Panel State >> Close", s=w330, f="") -> (s? t:f=w327:string)
            n107 = call <vilib>:"Add State(s) to Queue__jki_lib_state_machine.vi"("State(s) in Front (\"\")"="Data: Cleanup\nEvents: Unregister", "State(s) in (\"\")"="Process: Sync", "State(s) at Back (\"\")"="Exit") -> ("States Out"=w321:string)  [unwired: 12 in]
            n108 = call <vilib>:"Add State(s) to Queue__jki_lib_state_machine.vi"("State(s) in (\"\")"=w327, "State(s) at Back (\"\")"=w321) -> ("States Out"=w326:string)  [unwired: 13 in]
            n109 = call <vilib>:"Add State(s) to Queue__jki_lib_state_machine.vi"("State(s) in Front (\"\")"=w326, "State(s) in (\"\")"=w333) -> ("States Out"=w332:string)  [unwired: 13 in]
          }
          frame "---------- Process ----------" {
            # "Template Separator\n(You can make a copy of, or modify, this frame)"
            n110 = call <vilib>:"Add State(s) to Queue__jki_lib_state_machine.vi"("State(s) in (\"\")"=w338) -> ("States Out"=w337:string)  [unwired: 14 in]
          }
          frame "Process: Sync" {
            n111 = Unbundle By Name(w346) -> ("Self Reference"=w342:refnum<class "DisplayWaveforms.lvclass">)
            n112 = call <vilib>:"WaitOnProcessSync.vi"("error in (no error)"=w341, "SMO"=w342) -> ("error out"=w340:errorcluster, "Don't run?"=w345:bool)  [unwired: 7 in, 1 out]
            n113 = Select(t="Data: Cleanup\nEvents: Unregister\nExit", s=w345, f="") -> (s? t:f=w339:string)
            n114 = call <vilib>:"Add State(s) to Queue__jki_lib_state_machine.vi"("State(s) in Front (\"\")"=w339, "State(s) in (\"\")"=w349) -> ("States Out"=w348:string)  [unwired: 13 in]
          }
          frame "---------- Events ----------" {
            # "Template Separator\n(You can make a copy of, or modify, this frame)"
            n115 = call <vilib>:"Add State(s) to Queue__jki_lib_state_machine.vi"("State(s) in (\"\")"=w354) -> ("States Out"=w353:string)  [unwired: 14 in]
          }
          frame "Events: Register" {
            w361 = cluster{"New Value":refnum<user-event>} {"New Value"=refnum}  # Dependency.PublicEvents
            # "Get Event from SMO"
            # "Register for Data Producer Event here..."
            n116 = Unbundle By Name(w370) -> ("Self Reference"=w364:refnum<class "DisplayWaveforms.lvclass">)
            n117 = call <vilib>:"GetProtectedEvents.vi"("SMO"=w364) -> ("error out"=w359:errorcluster, "SMO Protected Events"=w368:T7)  [unwired: 8 in, 1 out]
            n118 = call "Chart[Template].GetProtectedEvents.vi"("DisplayWaveforms"=w364) -> ("error out"=w360:errorcluster, "Protected Events"=w365:T8)  [unwired: 8 in, 1 out]
            n119 = call "Chart[Template].GetDependencies.vi"("DisplayWaveforms"=w364) -> ("error out"=w358:errorcluster, "Dependencies"=w362:T9)  [unwired: 8 in, 1 out]
            n120 = Unbundle By Name(w362) -> ("New Value"=w357:refnum<user-event>)
            n121 = Not A Number/Path/Refnum?(number/path/refnum=w357) -> (NaN/Path/Refnum?=w356:bool)
            n122 = case shown="False" w356 {
              tunnel: w357 -> [w373 _]
              tunnel: w361 -> [w375 w378]
              tunnel: [w374 w377] -> w355
              frame False {
                n123 = Bundle By Name(cluster=w375, "New Value"=w373) -> (w374:cluster{"New Value":refnum<user-event>})
              }
              frame True {
                n124 = Bundle By Name(cluster=w378, "New Value"=refnum<user-event> refnum) -> (w377:cluster{"New Value":refnum<user-event>})
              }
            }
            n125 = register-events(w368, w365, w355) -> (reference out=w369:refnum<event-registration>, error out=w366:errorcluster)  [unwired: 2 in]
            n126 = Merge Errors(w363, w366, w358, w359, w360) -> (w367:errorcluster)
            n127 = call <vilib>:"Add State(s) to Queue__jki_lib_state_machine.vi"("State(s) in (\"\")"=w372) -> ("States Out"=w371:string)  [unwired: 14 in]
          }
          frame "Events: Unregister" {
            n128 = Unregister For Events(event registration refnum=w381, error in=w380) -> (error out=w379:errorcluster)
            n129 = call <vilib>:"Clear Errors.vi"("error in (no error)"=w379) -> ()  [unwired: 5 in, 2 out]
            n130 = call <vilib>:"Add State(s) to Queue__jki_lib_state_machine.vi"("State(s) in (\"\")"=w384) -> ("States Out"=w383:string)  [unwired: 14 in]
          }
          frame "---------- Action ----------" {
            n131 = call <vilib>:"Add State(s) to Queue__jki_lib_state_machine.vi"("State(s) in (\"\")"=w389) -> ("States Out"=w388:string)  [unwired: 14 in]
          }
          frame "Action: Clear Chart" {
            n132 = Unbundle By Name(w393) -> ("Self Reference"=w390:refnum<class "DisplayWaveforms.lvclass">)
            n133 = call-dynamic "Chart[Template].Clear.vi"("error in (no error)"=w392, "DisplayWaveforms"=w390) -> ("error out"=w391:errorcluster)  [unwired: 8 in, 1 out]
            n134 = call <vilib>:"Add State(s) to Queue__jki_lib_state_machine.vi"("State(s) in (\"\")"=w396) -> ("States Out"=w395:string)  [unwired: 14 in]
          }
          frame "Action: Export Chart" {
            # "Save snapshot of front panel"
            n135 = Unbundle By Name(w409) -> ("Self Reference"=w407:refnum<class "DisplayWaveforms.lvclass">, "Export Folder Path"=w400:path)
            n136 = call-dynamic "Chart[Template].Export.vi"("error in (no error)"=w408, "Export Folder Path"=w400, "DisplayWaveforms"=w407) -> ("error out"=w403:errorcluster)  [unwired: 7 in, 1 out]
            n137 = control-ref of="This VI"() -> (w406:refnum<vi>)
            n138 = invoke class="VI" method="FP.Get Image"(reference=w406, error in=w403, "visible area only"=TRUE ("Visible Area Only"), "image depth"=0 ("Image Depth")) -> (error out=w399:errorcluster, "image data"=w402:T10)  [unwired: 2 in, 4 out]
            n139 = Build Path(base path=w400, name or relative path=path "all_charts.png") -> (appended path=w401:path)
            n140 = call <vilib>:"Write PNG File.vi"("error in (no error)"=w399, "image data"=w402, "path to PNG file"=w401) -> ("error out"=w398:errorcluster)  [unwired: 7 in, 1 out]
            n141 = call <vilib>:"Add State(s) to Queue__jki_lib_state_machine.vi"("State(s) in (\"\")"=w412) -> ("States Out"=w411:string)  [unwired: 14 in]
          }
          frame "Action: SetChartParams" {
            n142 = Unbundle By Name(w417) -> ("Self Reference"=w414:refnum<class "DisplayWaveforms.lvclass">, "ChartParams"=w413:T4)
            n143 = call-dynamic "Chart[Template].SetParams.vi"("error in (no error)"=w416, "ChartParams"=w413, "DisplayWaveforms"=w414) -> ("error out"=w415:errorcluster)  [unwired: 7 in, 1 out]
            n144 = call <vilib>:"Add State(s) to Queue__jki_lib_state_machine.vi"("State(s) in (\"\")"=w420) -> ("States Out"=w419:string)  [unwired: 14 in]
          }
          frame "Action: Notify UI Closed" {
            # "Notify that the UI has been closed"
            n145 = Unbundle By Name(w423) -> ("Self Reference"=w424:refnum<class "DisplayWaveforms.lvclass">)
            n146 = call <vilib>:"Hide.vi"("error in (no error)"=w422, "SMO.UI"=w424) -> ("error out"=w421:errorcluster)  [unwired: 8 in, 1 out]
            n147 = call <vilib>:"Add State(s) to Queue__jki_lib_state_machine.vi"("State(s) in (\"\")"=w427) -> ("States Out"=w426:string)  [unwired: 14 in]
          }
        }
      }
    }
    frame Error {
    }
  }
  n148 = call-parent "Process.vi"("error in (no error)"=w8, "SMO.UI"=w7) -> ("error out"=w5:errorcluster, "SMO.UI out"=→"DisplayWaveforms out":refnum<class "DisplayWaveforms.lvclass">)  [unwired: 8 in]
  n149 = Merge Errors(w5, w4) -> (→"error out":errorcluster)
